vi "clone.vi"(0 "reference":refnum<class "RectangularNode.lvclass">, 5 "error in (no error)":errorcluster) -> (14 "reference out":refnum<class "RectangularNode.lvclass">, 15 "clonedRectanglularNode":refnum<class "AbstractNode.lvclass">, 19 "error out":errorcluster)   [LabVIEW 2012, in "RectangularNode.lvclass"]
doc: "public Object clone()"
uses:
  <resource>/Framework/Providers/Open_GDS/UML/RectangularNode_class/RectangularNode.lvclass
  <resource>/Framework/Providers/Open_GDS/UML/AbstractNode_class/AbstractNode.lvclass
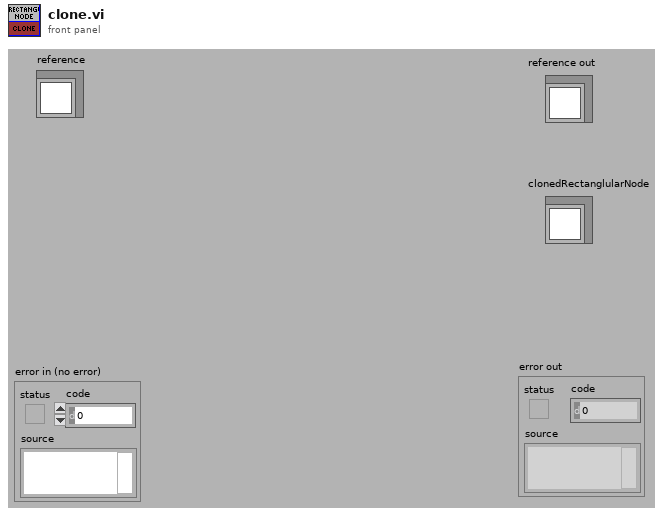
[diagram p1: front panel]
types:
  T1 = typedef "RectangularNode.lvclass/ObjectAttributes.ctl" = cluster{"Base class":T2, "bounds":T3}
  T2 = typedef "AbstractNode.lvclass/ObjectAttributes.ctl" = cluster{"parent":refnum<class "AbstractNode.lvclass">, "children":refnum<class "AbstractNode.lvclass">[], "Hidden":bool}
  T3 = typedef "Rectangle Rectangle2D.ctl" = cluster{"x":dbl, "y":dbl, "width":dbl, "height":dbl}
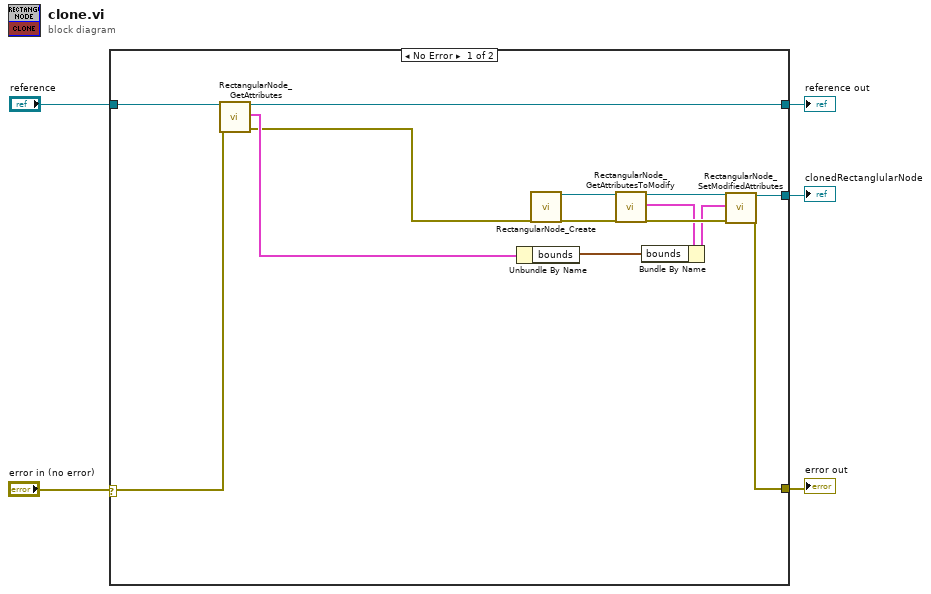
[diagram p0: block diagram]
diagram:
  n1 = case shown="No Error" "error in (no error)" {
    selector: "error in (no error)" -> [w17 w20]
    tunnel: "reference" -> [w19 w21]
    tunnel: [w18 w20] -> w4
    tunnel: [w6 w21] -> w3
    tunnel: [w16 _] -> w1
    frame No Error {
      n2 = call <resource>:"RectangularNode_GetAttributes.vi"("reference in"=w19, "error in (no error)"=w17) -> ("reference out"=w6:refnum<class "RectangularNode.lvclass">, "Attributes"=w15:T1, "error out"=w7:errorcluster)  [unwired: 15 out]
      n3 = Unbundle By Name(w15) -> ("bounds"=w10:T3)
      n4 = call <resource>:"RectangularNode_Create.vi"("error in (no error)"=w7) -> ("reference out"=w9:refnum<class "RectangularNode.lvclass">, "error out"=w8:errorcluster)  [unwired: 16 in, 1 out]
      n5 = call <resource>:"RectangularNode_GetAttributesToModify.vi"("reference in"=w9, "error in (no error)"=w8) -> ("reference out"=w13:refnum<class "RectangularNode.lvclass">, "Attributes"=w12:T1, "error out"=w14:errorcluster)  [unwired: 1 in, 14 out]
      n6 = Bundle By Name(cluster=w12, "bounds"=w10) -> (w11:T1)
      n7 = call <resource>:"RectangularNode_SetModifiedAttributes.vi"("reference in"=w13, "Attributes"=w11, "error in (no error)"=w14) -> ("reference out"=w16:refnum<class "RectangularNode.lvclass">, "error out"=w18:errorcluster)  [unwired: 3 in, 12 out]
    }
    frame Error {
    }
  }
  "reference out" <- w3
  "error out" <- w4
  "clonedRectanglularNode" <- w1
